vi "Insert Error Terminals.vi"(7 "grid multiplier (1)":i32=1, 8 "error in (no error)":errorcluster, 10 "case structure in":refnum<vi>, 11 "VI in":refnum<vi>) -> (0 "error out":errorcluster, 1 "error controls":cluster{"in":refnum<vi>, "out":refnum<vi>}, 2 "case structure out":refnum<vi>, 3 "VI out":refnum<vi>)   [LabVIEW 2017]
uses:
  <vilib>/Utility/miscctls.llb/LVPointTypeDef.ctl
  <resource>/dialog/lvconfig.llb/LV Config Read Numeric (I32).vi
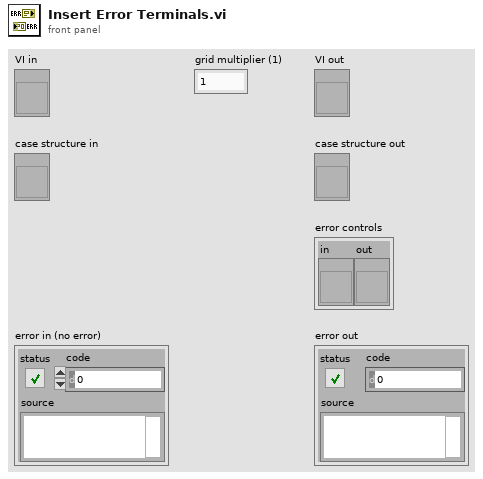
[diagram p1: front panel]
types:
  T1 = typedef "LVPointTypeDef.ctl" = cluster{"Horizontal":i16, "Vertical":i16}
  T2 = enum8{"Probe", "Diagram", "Panel Control", "3D Panel Control", "Dialog Panel Control", "Panel Indicator", "3D Panel Indicator", "Dialog Panel Indicator", "Power PC Control", "Power PC Indicator", "Silver Control", "Silver Indicator"}
  T3 = typedef "LVRectTypeDef.ctl" = cluster{"Left":i16, "Top":i16, "Right":i16, "Bottom":i16}
  T4 = cluster{"Left":i32, "Top":i32, "Right":i32, "Bottom":i32}
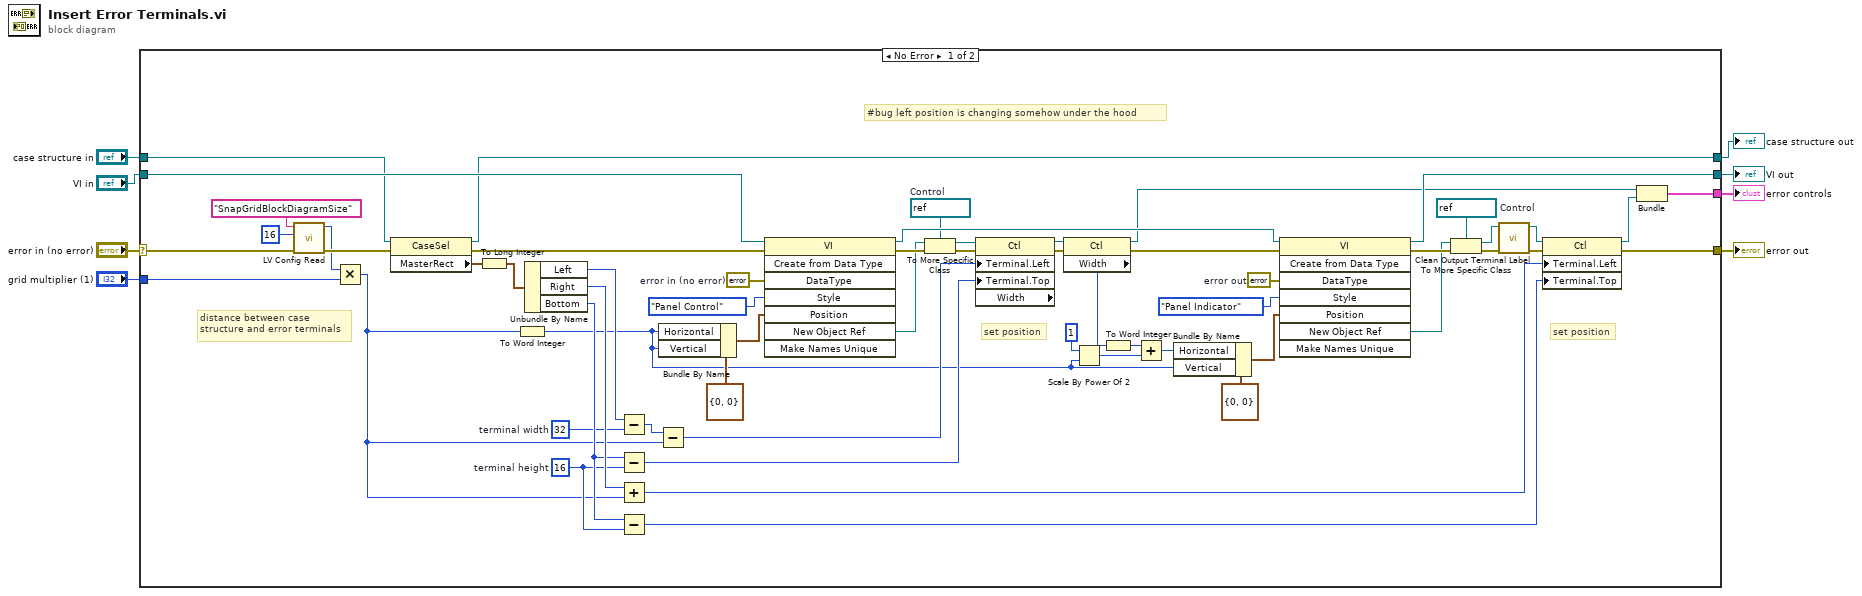
[diagram p0: block diagram]
diagram:
  n1 = case shown="No Error" "error in (no error)" {
    selector: "error in (no error)" -> [w24 w69]
    tunnel: "VI in" -> [w43 w68]
    tunnel: [w42 w69] -> w7
    tunnel: [w41 w68] -> w6
    tunnel: "case structure in" -> [w38 w67]
    tunnel: [w37 w67] -> w4
    tunnel: [w35 _] -> w3
    tunnel: "grid multiplier (1)" -> [w30 _]
    frame No Error {
      w25 = 16  # terminal height
      w26 = 32  # terminal width
      w50 = refnum<vi> refnum  # Control
      w55 = refnum<vi> refnum  # Control
      w58 = errorcluster {"status"=FALSE, "code"=0, "source"=""}  # error out
      w59 = errorcluster {"status"=FALSE, "code"=0, "source"=""}  # error in (no error)
      # "set position"
      # "set position"
      # "distance between case structure and error terminals"
      # "#bug left position is changing somehow under the hood"
      n2 = call-poly <resource>:"LV Config Read.vi"("error in"=w24, "default value"=i16 16, "key"="SnapGridBlockDiagramSize") -> ("error out"=w32:errorcluster, "value"=w31:i32)  [unwired: 2 in, 1 out]
      n3 = Multiply(x=w31, y=w30) -> (x*y=w13:i32)
      n4 = property class="CaseSel"(reference=w38, error in=w32) -> (reference out=w37:refnum<vi>, error out=w39:errorcluster, "MasterRect"=w40:T3)
      n5 = To Long Integer(number=w40) -> (32bit integer=w44:T4)
      n6 = To Word Integer(number=w13) -> (16bit integer=w11:i16)
      n7 = Unbundle By Name(w44) -> ("Left"=w65:i32, "Right"=w66:i32, "Bottom"=w64:i32)
      n8 = Subtract(x=w65, y=w26) -> (x-y=w29:i32)
      n9 = Subtract(x=w64, y=w25) -> (x-y=w47:i32)
      n10 = Add(x=w66, y=w13) -> (x+y=w28:i32)
      n11 = Subtract(x=w64, y=w25) -> (x-y=w51:i32)
      n12 = Subtract(x=w29, y=w13) -> (x-y=w27:i32)
      n13 = Bundle By Name(cluster=T1 {"Horizontal"=0, "Vertical"=0} ("Position"), "Horizontal"=w11, "Vertical"=w11) -> (w22:T1)
      n14 = invoke class="VI" method="Create from Data Type"(reference=w43, error in=w39, "DataType"=w59, "Style"=T2."Panel Control", "Position"=w22) -> (reference out=w60:refnum<vi>, error out=w63:errorcluster, "New Object Ref"=w49:refnum<vi>)  [unwired: 3 in, 5 out]
      n15 = To More Specific Class(target class=w50, reference=w49, error in=w63) -> (specific class reference=w48:refnum<vi>, error out=w45:errorcluster)
      n16 = property class="Ctl" props=["Terminal", "Left", "Terminal", "Top", "Width"](reference=w48, error in=w45, "Terminal.Left"=w27, "Terminal.Top"=w47) -> (reference out=w21:refnum<vi>, error out=w20:errorcluster)  [unwired: 1 out]
      n17 = property class="Ctl"(reference=w21, error in=w20) -> (reference out=w19:refnum<vi>, error out=w18:errorcluster, "Width"=w15:u32)
      n18 = Scale By Power Of 2(n=i16 1, x=w11) -> (x*2^n=w9:i16)
      n19 = To Word Integer(number=w15) -> (16bit integer=w12:i16)
      n20 = Add(x=w12, y=w9) -> (x+y=w14:i16)
      n21 = Bundle By Name(cluster=T1 {"Horizontal"=0, "Vertical"=0} ("Position"), "Horizontal"=w14, "Vertical"=w11) -> (w16:T1)
      n22 = invoke class="VI" method="Create from Data Type"(reference=w60, error in=w18, "DataType"=w58, "Style"=T2."Panel Indicator", "Position"=w16) -> (reference out=w41:refnum<vi>, error out=w62:errorcluster, "New Object Ref"=w56:refnum<vi>)  [unwired: 3 in, 5 out]
      n23 = To More Specific Class(target class=w55, reference=w56, error in=w62) -> (specific class reference=w54:refnum<vi>, error out=w53:errorcluster)
      n24 = call "Clean Output Terminal Label.vi"("error in (no error)"=w53, "control in"=w54) -> ("error out"=w46:errorcluster, "control out"=w52:refnum<vi>)  [unwired: 8 in]
      n25 = property class="Ctl"(reference=w52, error in=w46, "Terminal.Left"=w28, "Terminal.Top"=w51) -> (reference out=w36:refnum<vi>, error out=w42:errorcluster)
      n26 = Bundle(w19, "control out"=w36) -> (w35:cluster{refnum<vi>, "control out":refnum<vi>})  [unwired: 1 in]
    }
    frame Error {
    }
  }
  "error out" <- w7
  "VI out" <- w6
  "case structure out" <- w4
  "error controls" <- w3
